vi "Move parameters.vi"(2 "Current coordinates":cluster{"X":dbl, "Y":dbl, "Z":dbl}, 3 "Task":u16(ring) items=["MOVE", "HOME", "STOP", "Set Speed", "Info", "Set Zero", "MOVE2"], 4 "Speed":cluster{"Speed":i32, "Vi":i32, "Vi steps":i32}={"Speed"=3111, "Vi"=1000, "Vi steps"=800} {"Speed" min=50 max=8000 step=50 scale=50.0..8000.0}, 5 "X0":T3={"X (um)"=1000.0, "X 2"=FALSE, "Y (um)"=0.0, "Y 2"=FALSE, "Z (um)"=0.0, "Z 2"=FALSE} {"X (um)" step=1.0}, 6 "PosCtrl":T1={"Go x"=FALSE, "Back x"=FALSE, "Go y"=FALSE, "Back y"=FALSE, "Go z"=FALSE, "Back z"=FALSE, "dX (um)"=1000.0, "dY (um)"=0.0, "dZ (um)"=0.0} {"dX (um)" step=1.0}, 7 "Scaling":cluster{"X":u16, "Y":u16, "Z":u16} {"Z" items=["X", "Z", "None"]; "Y" items=["X", "Z", "None"]; "X" items=["X", "Z", "None"]}) -> (0 "PosCtrl out":T1={"Go x"=FALSE, "Back x"=FALSE, "Go y"=FALSE, "Back y"=FALSE, "Go z"=FALSE, "Back z"=FALSE, "dX (um)"=1000.0, "dY (um)"=0.0, "dZ (um)"=0.0} {"dX (um)" step=1.0}, 1 "Move info":T2={"Task 2"=0, "Position to go 2"={"Position"={"X"=FALSE, "Target X (um)"=1000.0, "Current X (um)"=1000.0, "Scaling X"=0, "Y"=FALSE, "Target Y (um)"=0.0, "Current Y (um)"=0.0, "Scaling Y"=0, "Z"=FALSE, "Target Z (um)"=0.0, "Current Z (um)"=0.0, "Scaling Z"=0}, "Speed"={"Speed"=3111, "Vi steps"=800, "Vi"=1000}}} {"Task 2" items=["MOVE", "HOME", "STOP", "Set Speed", "Info", "Set Zero", "MOVE2"]; "Position to go 2"."Speed"."Speed" min=50 max=8000 step=50 scale=50.0..8000.0; "Position to go 2"."Position"."Current X (um)" step=1.0; "Position to go 2"."Position"."Scaling Z" items=["X", "Z", "None"]; "Position to go 2"."Position"."Scaling Y" items=["X", "Z", "None"]; "Position to go 2"."Position"."Scaling X" items=["X", "Z", "None"]; "Position to go 2"."Position"."Target X (um)" step=1.0})   [LabVIEW 2014]
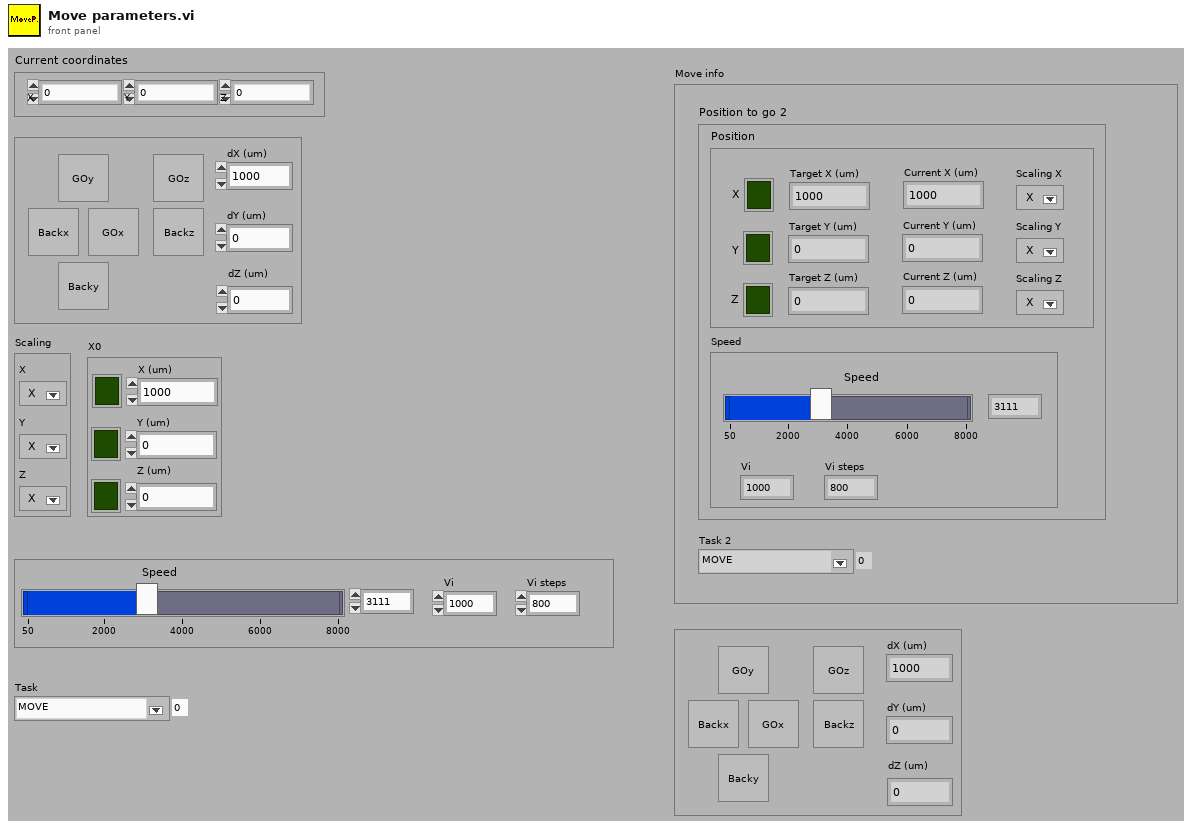
[diagram p1: front panel]
types:
  T1 = cluster{"Go x":bool, "Back x":bool, "Go y":bool, "Back y":bool, "Go z":bool, "Back z":bool, "dX (um)":dbl, "dY (um)":dbl, "dZ (um)":dbl}
  T2 = cluster{"Task 2":u16, "Position to go 2":cluster{"Position":cluster{"X":bool, "Target X (um)":dbl, "Current X (um)":dbl, "Scaling X":u16, "Y":bool, "Target Y (um)":dbl, "Current Y (um)":dbl, "Scaling Y":u16, "Z":bool, "Target Z (um)":dbl, "Current Z (um)":dbl, "Scaling Z":u16}, "Speed":cluster{"Speed":i32, "Vi steps":i32, "Vi":i32}}}
  T3 = cluster{"X (um)":dbl, "X 2":bool, "Y (um)":dbl, "Y 2":bool, "Z (um)":dbl, "Z 2":bool}
  T4 = cluster{bool, dbl, "X":dbl, "X":u16, bool, dbl, "Y":dbl, "Y":u16, bool, dbl, "Z":dbl, "Z":u16}
  T5 = cluster{cluster{bool, dbl, "X":dbl, "X":u16, bool, dbl, "Y":dbl, "Y":u16, bool, dbl, "Z":dbl, "Z":u16}, "Speed":cluster{"Speed":i32, "Vi":i32, "Vi steps":i32}}
  T6 = cluster{"Task":u16, cluster{cluster{bool, dbl, "X":dbl, "X":u16, bool, dbl, "Y":dbl, "Y":u16, bool, dbl, "Z":dbl, "Z":u16}, "Speed":cluster{"Speed":i32, "Vi":i32, "Vi steps":i32}}}
  T7 = cluster{bool, "X (um)":dbl, "X":dbl, "X":u16, bool, "Y (um)":dbl, "Y":dbl, "Y":u16, bool, "Z (um)":dbl, "Z":dbl, "Z":u16}
  T8 = cluster{cluster{bool, "X (um)":dbl, "X":dbl, "X":u16, bool, "Y (um)":dbl, "Y":dbl, "Y":u16, bool, "Z (um)":dbl, "Z":dbl, "Z":u16}, "Speed":cluster{"Speed":i32, "Vi":i32, "Vi steps":i32}}
  T9 = cluster{"Task":u16, cluster{cluster{bool, "X (um)":dbl, "X":dbl, "X":u16, bool, "Y (um)":dbl, "Y":dbl, "Y":u16, bool, "Z (um)":dbl, "Z":dbl, "Z":u16}, "Speed":cluster{"Speed":i32, "Vi":i32, "Vi steps":i32}}}
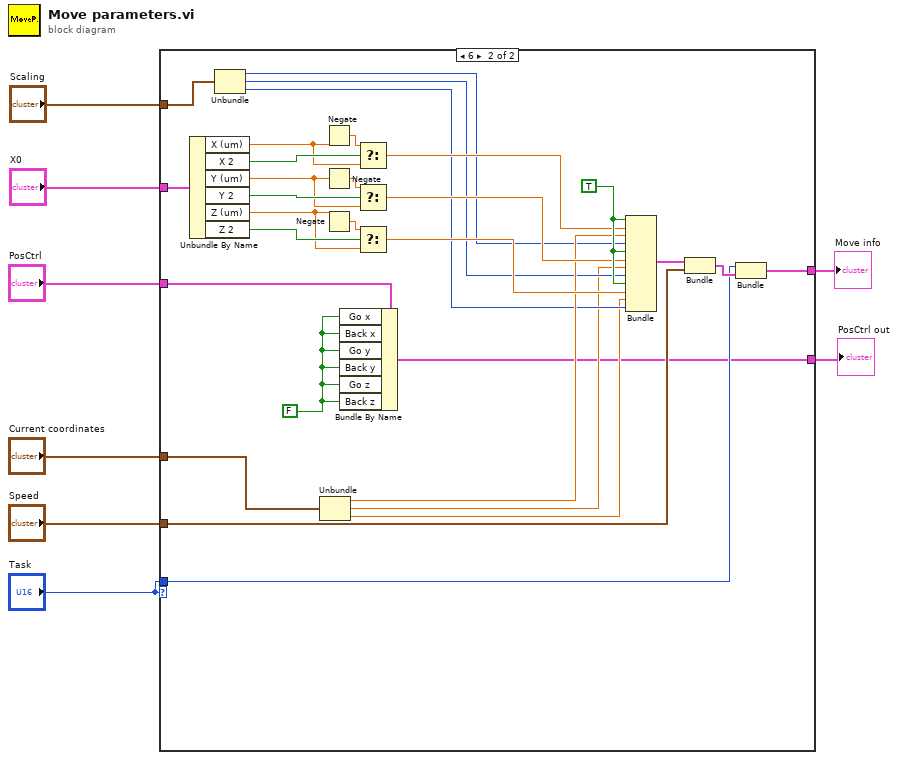
[diagram p0: block diagram]
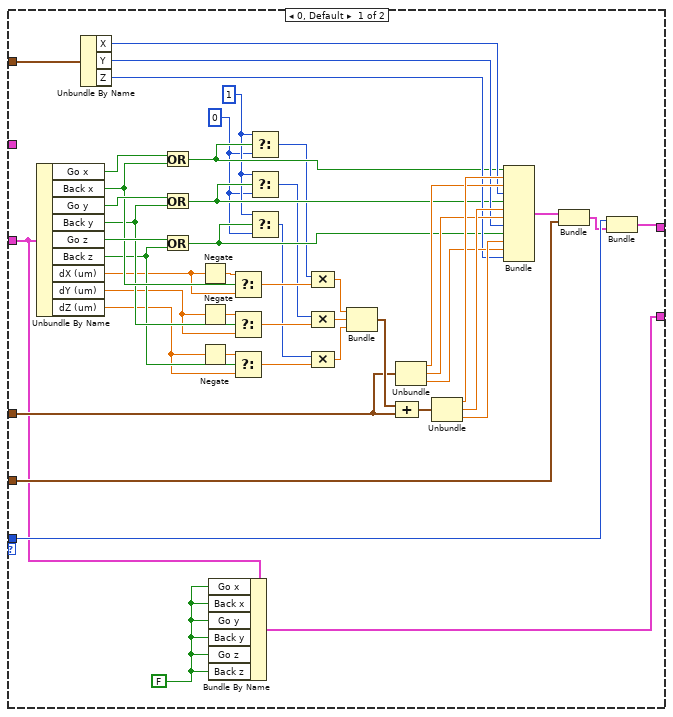
[diagram p2: hidden frame]
diagram:
  n1 = case shown="6" "Task" {
    tunnel: "Speed" -> [w26 w62]
    tunnel: "PosCtrl" -> [w21 w58]
    tunnel: "Current coordinates" -> [w35 w71]
    tunnel: "Scaling" -> [w31 w69]
    tunnel: [w23 w60] -> w2
    tunnel: "X0" -> [_ w81]
    tunnel: "Task" -> [w25 w59]
    tunnel: [w20 w57] -> w1
    frame 0, Default {
      w22 = FALSE
      w12 = 0 ("f")
      w13 = 1
      n2 = Unbundle By Name(w21) -> ("Go x"=w55:bool, "Back x"=w50:bool, "Go y"=w54:bool, "Back y"=w49:bool, "Go z"=w53:bool, "Back z"=w48:bool, "dX (um)"=w44:dbl, "dY (um)"=w43:dbl, "dZ (um)"=w42:dbl)
      n3 = Unbundle By Name(w31) -> ("X"=w30:u16, "Y"=w29:u16, "Z"=w28:u16)
      n4 = Or(x=w55, y=w50) -> (x .or. y?=w16:bool)
      n5 = Or(x=w54, y=w49) -> (x .or. y?=w15:bool)
      n6 = Or(x=w53, y=w48) -> (x .or. y?=w14:bool)
      n7 = Negate(x=w44) -> (-x=w47:dbl)
      n8 = Negate(x=w43) -> (-x=w46:dbl)
      n9 = Negate(x=w42) -> (-x=w45:dbl)
      n10 = Bundle By Name(cluster=w21, "Go x"=w22, "Back x"=w22, "Go y"=w22, "Back y"=w22, "Go z"=w22, "Back z"=w22) -> (w20:T1)
      n11 = Select(t=w47, s=w50, f=w44) -> (s? t:f=w41:dbl)
      n12 = Select(t=w46, s=w49, f=w43) -> (s? t:f=w40:dbl)
      n13 = Select(t=w45, s=w48, f=w42) -> (s? t:f=w39:dbl)
      n14 = Select(t=w13, s=w16, f=w12) -> (s? t:f=w11:i32)
      n15 = Select(t=w13, s=w15, f=w12) -> (s? t:f=w10:i32)
      n16 = Select(t=w13, s=w14, f=w12) -> (s? t:f=w9:i32)
      n17 = Compound Arithmetic op=MULTIPLY(w11, w41) -> (w19:dbl)
      n18 = Compound Arithmetic op=MULTIPLY(w10, w40) -> (w18:dbl)
      n19 = Compound Arithmetic op=MULTIPLY(w9, w39) -> (w17:dbl)
      n20 = Bundle(w19, w18, w17) -> (w52:cluster{dbl, dbl, dbl})  [unwired: 1 in]
      n21 = Unbundle(w35) -> ("X"=w34:dbl, "Y"=w33:dbl, "Z"=w32:dbl)
      n22 = Compound Arithmetic op=ADD(w52, w35) -> (w51:cluster{dbl, dbl, dbl})
      n23 = Unbundle(w51) -> (w38:dbl, w37:dbl, w36:dbl)
      n24 = Bundle(w16, w38, "X"=w34, "X"=w30, w15, w37, "Y"=w33, "Y"=w29, w14, w36, "Z"=w32, "Z"=w28) -> (w27:T4)  [unwired: 1 in]
      n25 = Bundle(w27, "Speed"=w26) -> (w24:T5)  [unwired: 1 in]
      n26 = Bundle("Task"=w25, w24) -> (w23:T6)  [unwired: 1 in]
    }
    frame 6 {
      w56 = FALSE
      w85 = TRUE
      n27 = Unbundle By Name(w81) -> ("X (um)"=w77:dbl, "X 2"=w80:bool, "Y (um)"=w76:dbl, "Y 2"=w79:bool, "Z (um)"=w75:dbl, "Z 2"=w78:bool)
      n28 = Unbundle(w69) -> ("X"=w68:u16, "Y"=w67:u16, "Z"=w66:u16)
      n29 = Unbundle(w71) -> ("X"=w70:dbl, "Y"=w64:dbl, "Z"=w65:dbl)
      n30 = Negate(x=w77) -> (-x=w84:dbl)
      n31 = Negate(x=w76) -> (-x=w83:dbl)
      n32 = Negate(x=w75) -> (-x=w82:dbl)
      n33 = Bundle By Name(cluster=w58, "Go x"=w56, "Back x"=w56, "Go y"=w56, "Back y"=w56, "Go z"=w56, "Back z"=w56) -> (w57:T1)
      n34 = Select(t=w84, s=w80, f=w77) -> (s? t:f=w74:dbl)
      n35 = Select(t=w83, s=w79, f=w76) -> (s? t:f=w73:dbl)
      n36 = Select(t=w82, s=w78, f=w75) -> (s? t:f=w72:dbl)
      n37 = Bundle(w85, "X (um)"=w74, "X"=w70, "X"=w68, w85, "Y (um)"=w73, "Y"=w64, "Y"=w67, w85, "Z (um)"=w72, "Z"=w65, "Z"=w66) -> (w63:T7)  [unwired: 1 in]
      n38 = Bundle(w63, "Speed"=w62) -> (w61:T8)  [unwired: 1 in]
      n39 = Bundle("Task"=w59, w61) -> (w60:T9)  [unwired: 1 in]
    }
  }
  "Move info" <- w2
  "PosCtrl out" <- w1
